vi "signalAcquisition.vi"(8 "Error IN":errorcluster caption="constante d'erreur", 10 "mainConfigs":T1={"spectroConfig"={"Grating"=0, "waveLength"=0, "sampleTime"=0.0, "nbStrip"=0, "gap"=0, "Background path"=path "", "temperature"=0.0, "binning"=0, "Camera handle"=0, "Spectro handle"=0, "Xdim"=0, "Ydim"=0}, "tempConfig"={"ComPort"="COM4", "SensorNumber"=1.0, "PID"={"P"=0.0, "I"=0.0, "D"=0.0}}, "expConfig"={"colorParameters"={"giver"="", "acceptor"=[]}, "recordDataInTDMS?"=TRUE, "PID_mode"=enum."rampe"}}, 11 "Répertoire de sortie du fichier TDMS":path=path "") -> (0 "Error OUT":errorcluster caption="constante d'erreur", 2 "tempData":i32[](array[numeric]), 3 "spectroData":i32[][](array[numeric]))   [LabVIEW 2020]
uses:
  defTypeConfigs/mainConfigs.ctl
  defTypeConfigs/spectroConfig.ctl
  defTypeConfigs/tempConfig.ctl
  defTypeConfigs/expConfig.ctl
panel:
  out "readyToStart?":bool
  out "Noms voies TDMS":string[](array[string])
  out "TDMS output file path":path
  out "fichier tdms en sortie":refnum<k34>
  in  "Stop acquisition":bool
  # "GET DATAS \nFROM SPECTROMETER"
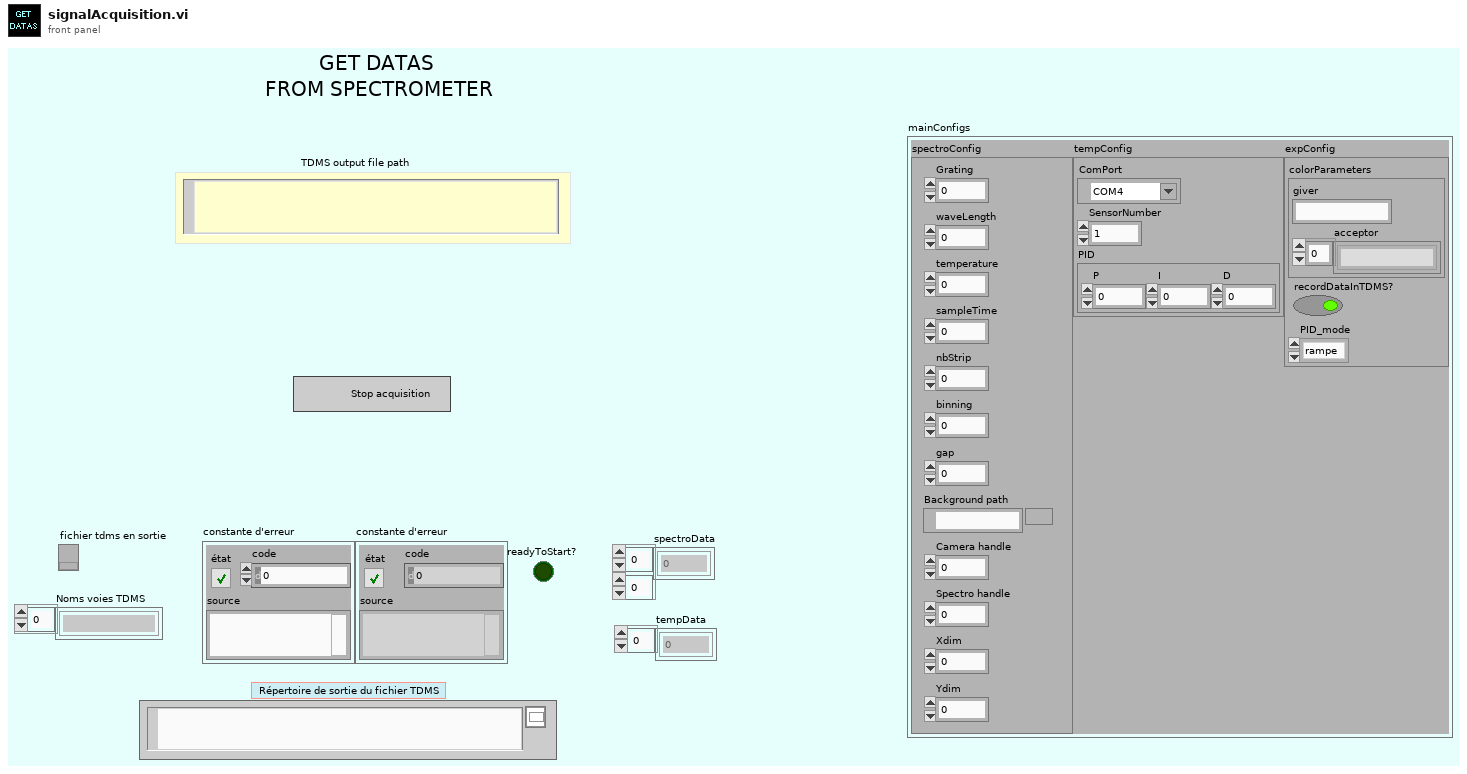
[diagram p1: front panel]
types:
  T1 = typedef "mainConfigs.ctl" = cluster{"spectroConfig":T2, "tempConfig":T3, "expConfig":T4}
  T2 = typedef "spectroConfig.ctl" = cluster{"Grating":i32, "waveLength":i32, "sampleTime":dbl, "nbStrip":i32, "gap":i32, "Background path":path, "temperature":dbl, "binning":i32, "Camera handle":i32, "Spectro handle":i32, "Xdim":i32, "Ydim":i32}
  T3 = typedef "tempConfig.ctl" = cluster{"ComPort":refnum<visa-resource-name>, "SensorNumber":dbl, "PID":cluster{"P":dbl, "I":dbl, "D":dbl}}
  T4 = typedef "expConfig.ctl" = cluster{"colorParameters":cluster{"giver":string, "acceptor":string[]}, "recordDataInTDMS?":bool, "PID_mode":enum16{"rampe", "triangle", "sinus", "carré", "continu"}}
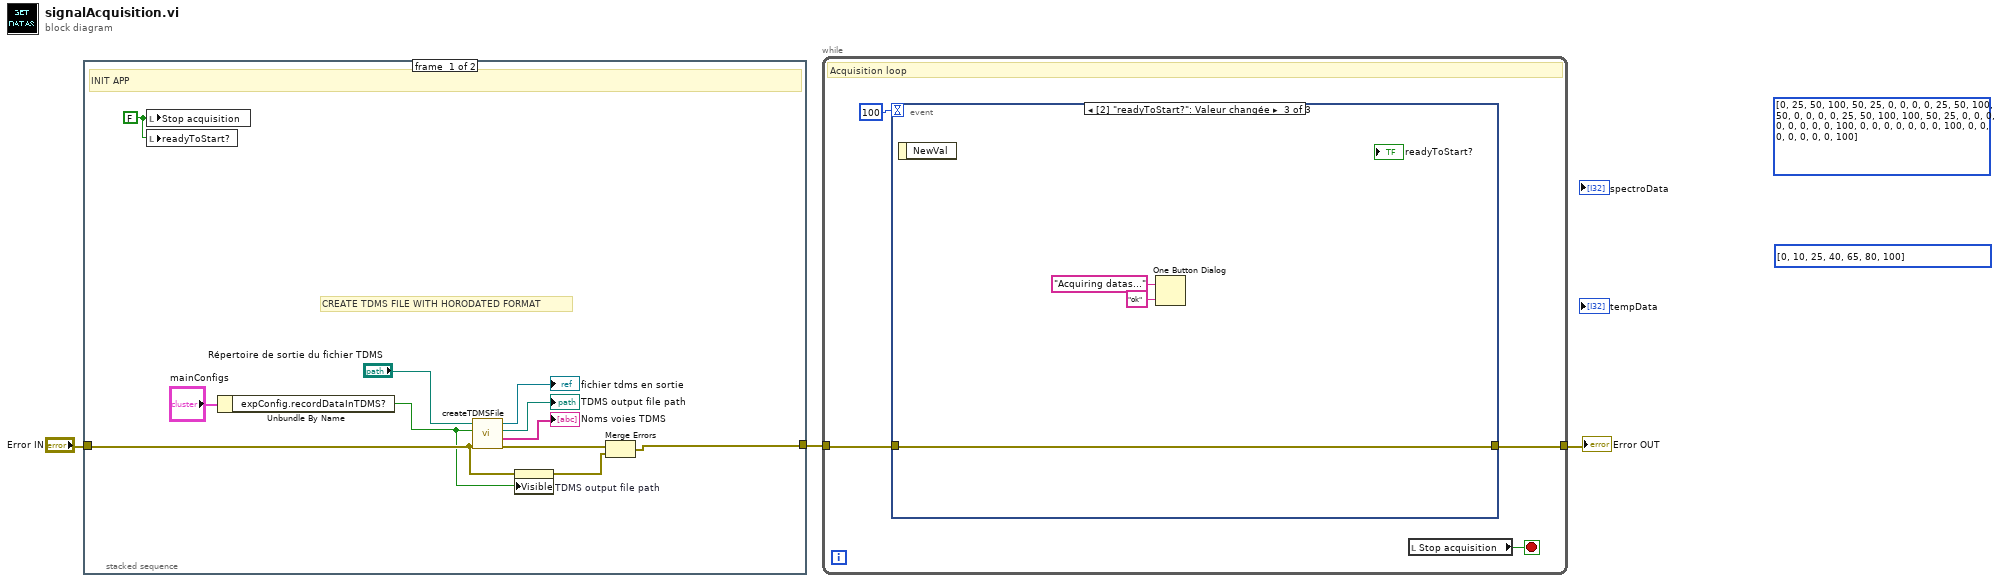
[diagram p0: block diagram]
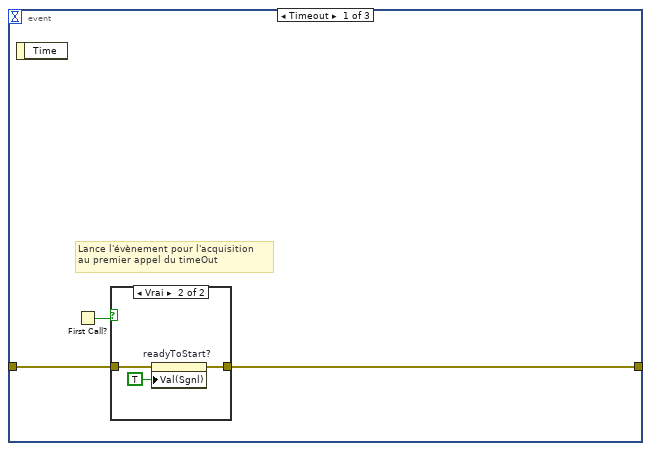
[diagram p3: hidden frame]
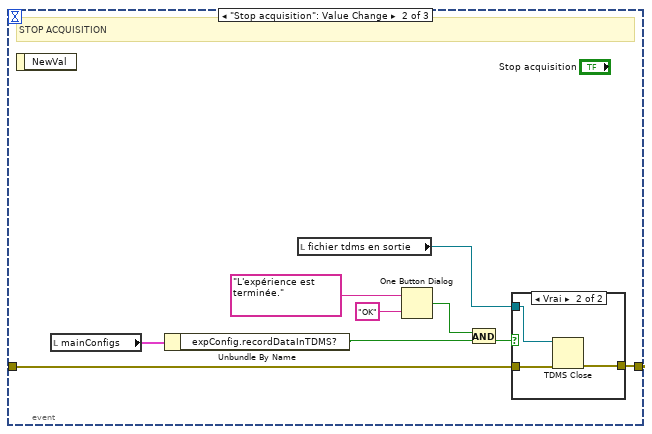
[diagram p5: hidden frame]
diagram:
  (unwired) i32[] [0, 10, 25, 40, 65, 80, 100]
  (unwired) i32[][] [[0, 25, 50, 100, 50, 25, 0], [0, 0, 0, 25, 50, 100, 50], [0, 0, 0, 0, 25, 50, 100], [100, 50, 25, 0, 0, 0, 0], [0, 0, 0, 0, 100, 0, 0], [0, 0, 0, 0, 0, 100, 0], [0, 0, 0, 0, 0, 0, 100]]
  n1 = stacked-sequence {
    tunnel: "Error IN" -> [w10 _]
    tunnel: [w5 _] -> w1
    frame #0 {
      w4 = FALSE ("Stop acquisition")
      # "CREATE TDMS FILE WITH HORODATED FORMAT"
      # "INIT APP"
      n2 = local write "Stop acquisition"(w4) -> ()
      n3 = local write "readyToStart?"(w4) -> ()
      n4 = Unbundle By Name("mainConfigs") -> ("expConfig.recordDataInTDMS?"=w7:bool)
      n5 = call "createTDMSFile.vi"("Error IN"=w10, "TDMS bool"=w7, "Répertoire de sortie du fichier TDMS"="Répertoire de sortie du fichier TDMS") -> ("Error OUT"=w9:errorcluster, "Noms voies TDMS"=→"Noms voies TDMS":string[], "Chemin de sortie TDMS"=→"TDMS output file path":path, "fichier tdms en sortie"=→"fichier tdms en sortie":refnum<k34>)  [unwired: 5 in]
      n6 = property on="TDMS output file path" class="Chm"(error in=w10, "Visible"=w7) -> (error out=w8:errorcluster)  [unwired: 1 in, 1 out]
      n7 = Merge Errors(w9, w8) -> (w5:errorcluster)
    }
    frame #1 {
    }
  }
  n8 = while {
    tunnel: [w16] -> w3
    tunnel: w1 -> [w17]
    stop <- w15 stop-if-true
    # "Acquisition loop"
    n9 = event shown="[2] \"readyToStart?\": Valeur changée" {
      selector: _ -> [_ _ _]
      dyn-events: _ -> [_ _ _]
      timeout: 100 -> [_ _ _]
      tunnel: w17 -> [w20 w34 w41]
      tunnel: [w19 w33 w41] -> w16
      event Timeout {
        # "Lance l'évènement pour l'acquisition\nau premier appel du timeOut"
        n10 = event-data() -> ()  [unwired: 1 in, 1 out]
        n11 = First Call?() -> (First Call?: T/F=w21:bool)
        n12 = case shown="Vrai" w21 {
          tunnel: w20 -> [w22 w24]
          tunnel: [w22 w23] -> w19
          frame False {
          }
          frame True {
            n13 = property on="readyToStart?" class="Bool (strict)"(error in=w24, "Val(Sgnl)"=TRUE ("Valeur (Signalisation)")) -> (error out=w23:errorcluster)  [unwired: 1 in, 1 out]
          }
        }
      }
      event "Stop acquisition": Value Change {
        # "STOP ACQUISITION"
        n14 = event-data() -> ()  [unwired: 1 in, 1 out]
        n15 = local read "mainConfigs"() -> (w26:T1)
        n16 = Unbundle By Name(w26) -> ("expConfig.recordDataInTDMS?"=w27:bool)
        n17 = local read "fichier tdms en sortie"() -> (w28:refnum<k34>)
        n18 = One Button Dialog(message="L'expérience est terminée.", button name ("OK")="OK" ("nom du bouton (\"OK\")")) -> (true=w29:bool)
        n19 = And(x=w29, y=w27) -> (x .and. y?=w30:bool)
        n20 = case shown="Vrai" w30 {
          tunnel: w34 -> [w35 w38]
          tunnel: [w35 w37] -> w33
          tunnel: w28 -> [_ w36]
          frame False {
          }
          frame True {
            n21 = TDMS Close(8:w38, 11:w36) -> (0:w37:errorcluster)  [unwired: 1 out]
          }
        }
      }
      event "readyToStart?": Value Change {
        n22 = event-data() -> ()  [unwired: 1 in, 1 out]
        n23 = One Button Dialog(message="Acquiring datas...", button name ("OK")="ok" ("nom du bouton (\"OK\")")) -> ()  [unwired: 1 out]
      }
    }
    n24 = local read "Stop acquisition"() -> (w15:bool)
  }
  "Error OUT" <- w3
